vi "Write output.vi"(10 "output":dbl format="%.2f", 11 "PID Output Rate Limiter in":refnum<class "PID Output Rate Limiter.lvclass">) -> (3 "PID Output Rate Limiter out":refnum<class "PID Output Rate Limiter.lvclass">)   [LabVIEW 2019, in "control.lvlib" / "PID Output Rate Limiter.lvclass"]
uses:
  PID Output Rate Limiter.lvclass
  PID Output Rate Limiter.lvclass/PID Output Rate Limiter.ctl
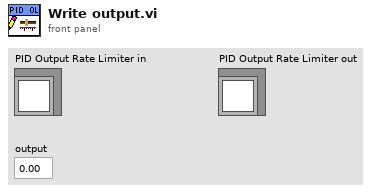
[diagram p1: front panel]
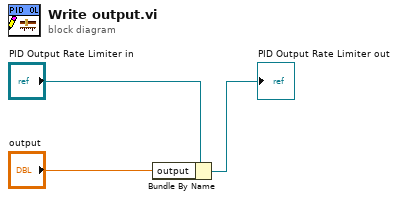
[diagram p0: block diagram]
diagram:
  n1 = Bundle By Name(cluster="PID Output Rate Limiter in", "output"="output") -> (→"PID Output Rate Limiter out":refnum<class "PID Output Rate Limiter.lvclass">)
